vi "Write FPGA Reference.vi"(8 "error in (no error)":errorcluster, 10 "FPGA Reference.lvclass":refnum<class "FPGA Reference.lvclass">, 11 "System Modules Factory in":refnum<class "System Modules Factory.lvclass">) -> (0 "error out":errorcluster, 3 "System Modules Factory out":refnum<class "System Modules Factory.lvclass">)   [LabVIEW 2019, in "System Modules Factory.lvclass"]
uses:
  System Modules Factory.lvclass
  SPIM Library/Hardware Actors/Parents/FPGA Reference/FPGA Reference.lvclass
  System Modules Factory.lvclass/System Modules Factory.ctl
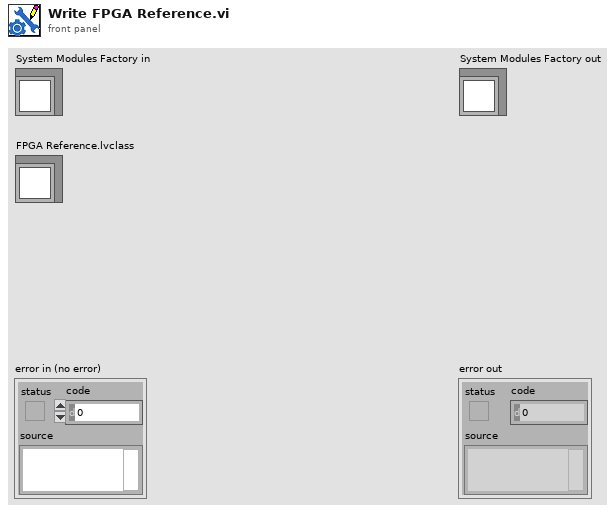
[diagram p1: front panel]
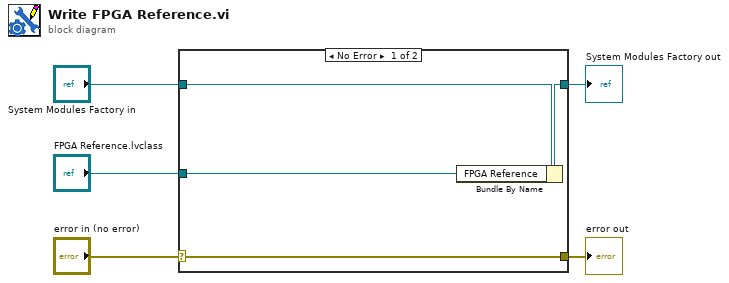
[diagram p0: block diagram]
diagram:
  n1 = case shown="No Error" "error in (no error)" {
    selector: "error in (no error)" -> [w9 w10]
    tunnel: [w9 w10] -> w4
    tunnel: [w7 w11] -> w2
    tunnel: "System Modules Factory in" -> [w8 w11]
    tunnel: "FPGA Reference.lvclass" -> [w6 _]
    frame No Error {
      n2 = Bundle By Name(cluster=w8, "FPGA Reference"=w6) -> (w7:refnum<class "System Modules Factory.lvclass">)
    }
    frame Error {
    }
  }
  "error out" <- w4
  "System Modules Factory out" <- w2
